vi "PositionReceiverAngleAttacker.vi"(6 "AnguloGol":dbl, 8 "error in (no error)":errorcluster, 9 "atacando contra":bool, 10 "Game":refnum<class "Game.lvclass">, 11 "PositionToReceivePassSkill in":refnum<class "PositionToReceivePassSkill.lvclass">) -> (0 "error out":errorcluster, 1 "AttackerPositive?":bool, 2 "theta final":dbl, 3 "PositionToReceivePassSkill out":refnum<class "PositionToReceivePassSkill.lvclass">, 4 "YdoAttacker 2":dbl, 5 "XdoAttacker 2":dbl)   [LabVIEW 2018, in "PositionToReceivePassSkill.lvclass"]
uses:
  PositionToReceivePassSkill.lvclass
  Game_class/Game.lvclass
  Game_class/Game.lvclass/Game.ctl
  Team_class/Team.lvclass/Team.ctl
  Robot_class/roles.ctl
  Robot_class/Robot.lvclass/Robot.ctl
  Object_class/Object.lvclass/Object.ctl
  Robot_class/Read role.vi
  Object_class/Read x.vi
  Object_class/Read y.vi
  Robot_class/Read id.vi
  Game_class/Read OffensiveTeam.vi
  Game_class/Read EnemyRef.vi
  Game_class/Read FieldRef.vi
  Team_class/Read RobotRef.vi
  Enemy_class/Enemy.lvclass
  Ally_class/Ally.lvclass
  Robot_class/Robot.lvclass
  Field_class/Field.lvclass
panel:
  in  "valor de theta 3":dbl
  in  "tamanho do intervalo 3":dbl
  in  "inicio do intervalo 3":dbl
  in  "fim do intervalo 3":dbl
  in  "Contador 4":dbl
  in  "Array 3":dbl[](array[numeric])=[0.0, 0.0, 0.0, 0.0, 0.0, 0.0]
  in  "valor de theta 2":dbl
  in  "tamanho do intervalo 2":dbl
  in  "inicio do intervalo 2":dbl
  in  "fim do intervalo 2":dbl
  in  "Contador 3":dbl
  in  "Array 2":dbl[](array[numeric])=[0.0, 0.0, 0.0, 0.0, 0.0, 0.0]
  in  "XdoAttacker":dbl
  in  "YdoAttacker":dbl
  in  "RobôsParaAnalisar":dbl[][](array[numeric])=[[99999.0, 99999.0], [99999.0, 99999.0], [99999.0, 99999.0], [99999.0, 99999.0], [99999.0, 99999.0], [99999.0, 99999.0], [99999.0, 99999.0]]
  in  "Contador":dbl
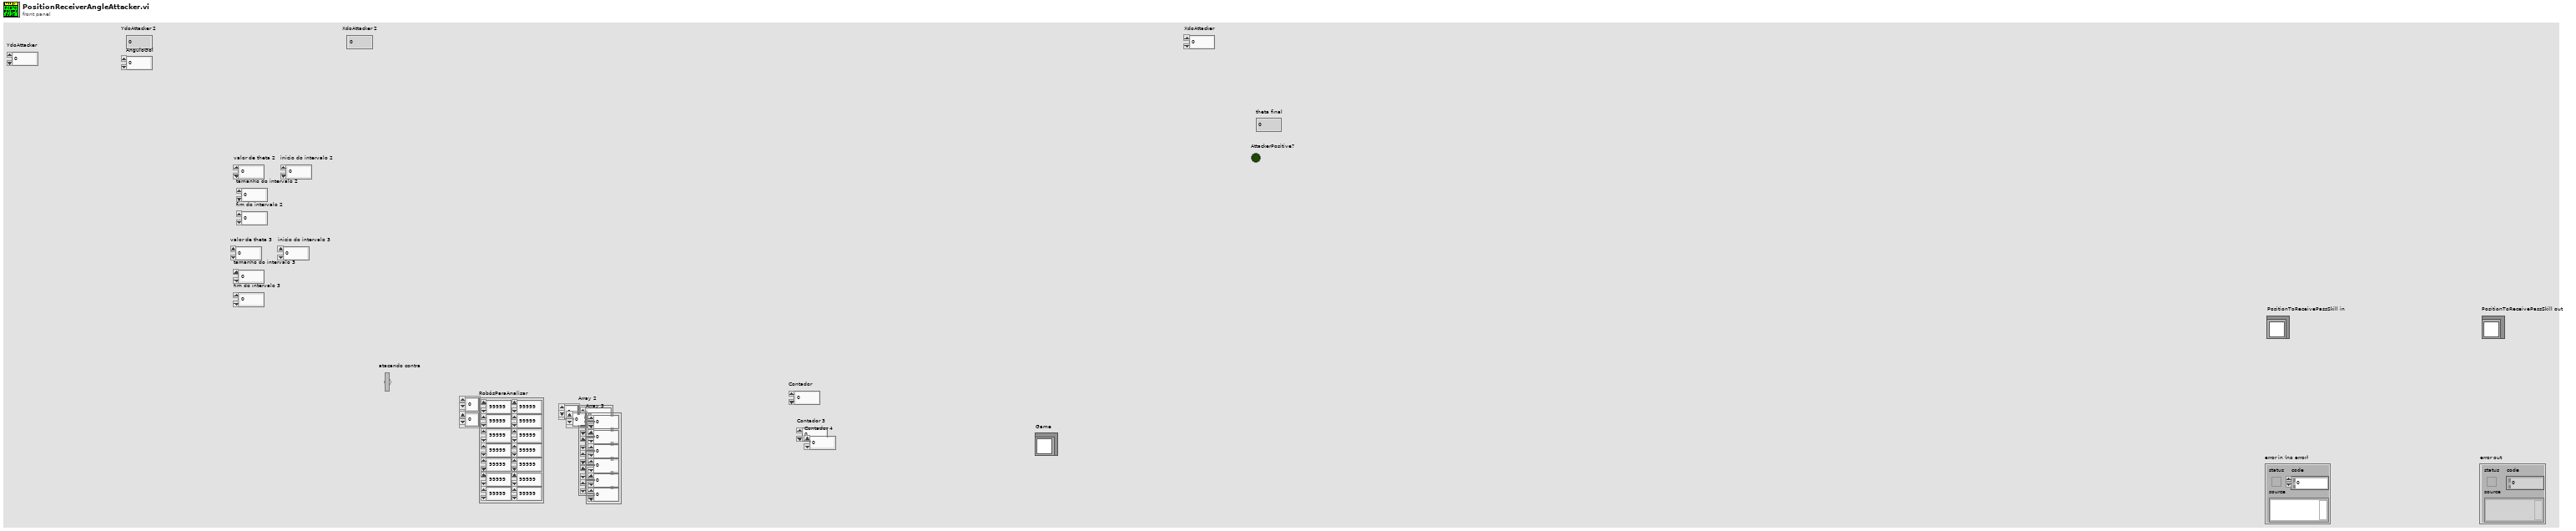
[diagram p1: front panel]
types:
  T1 = typedef "roles.ctl" = enum16{"PenaltyDefense", "PreparePassReceiver", "PassObserver", "Timeout", "Goto", "ZigZag", "None", "BallOutOfField", "DefenderArea", "Duelist", "AttackerStop", "FollowAttacker", "KeeperRole", "KickPenalty", "AttackerAimGoal", "AttackerBlock", "Marker", "Halt", "Shoot", "PassKicker", "PassReceiver", "TestRole", "PenaltyAttacker"}
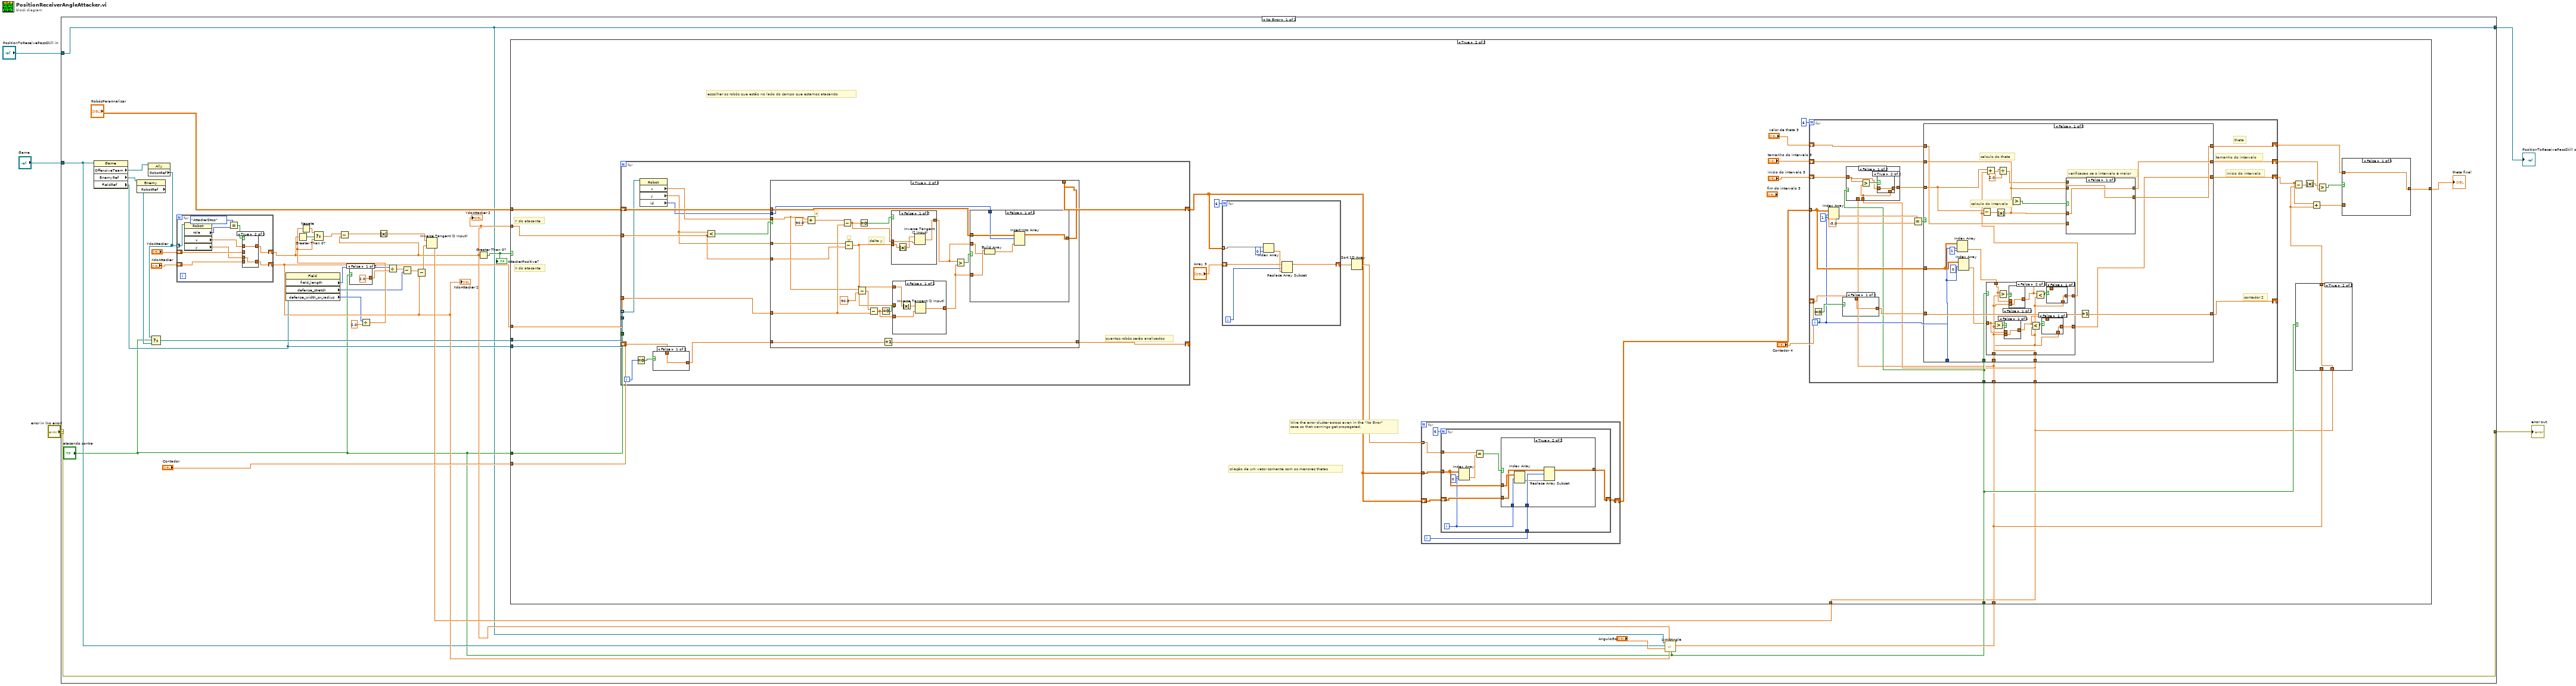
[diagram p0: block diagram]
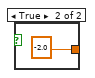
[diagram p2: hidden frame]
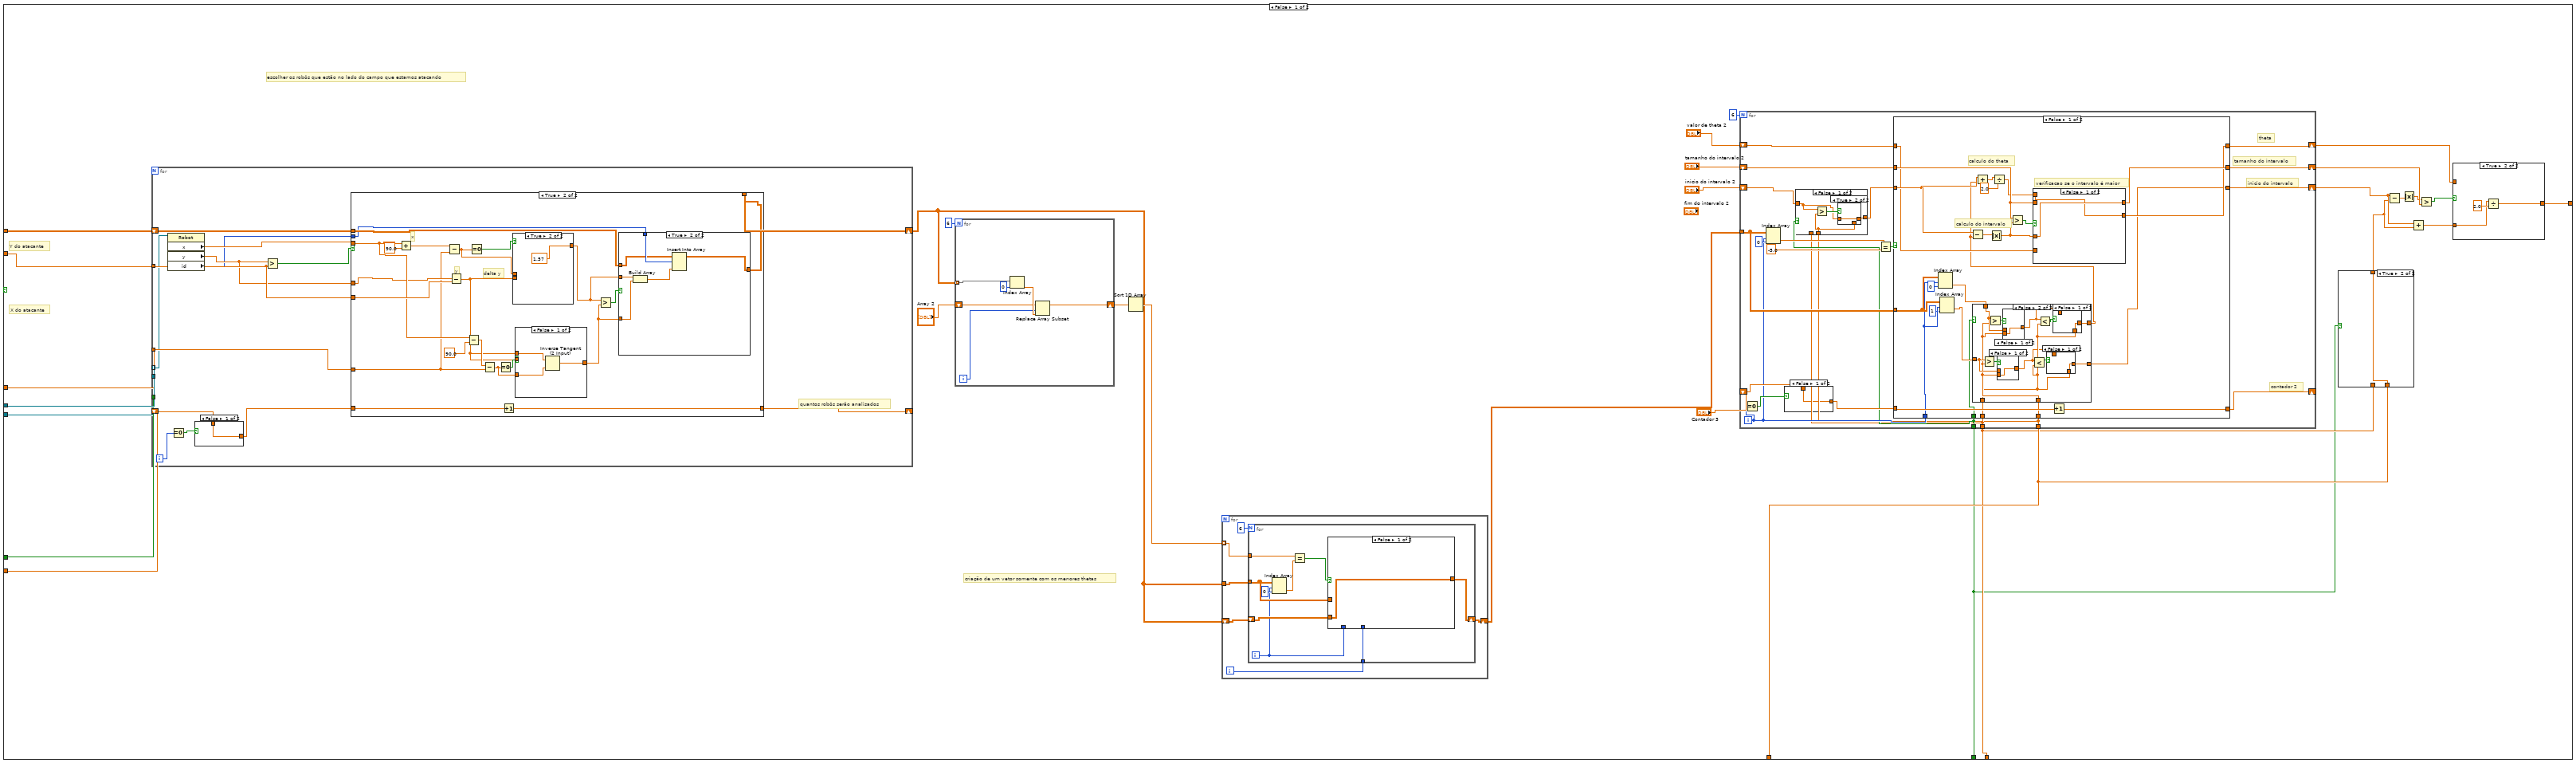
[diagram p3: hidden frame]
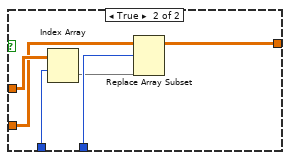
[diagram p6: hidden frame]
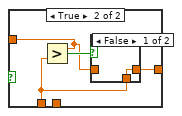
[diagram p8: hidden frame]
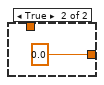
[diagram p10: hidden frame]
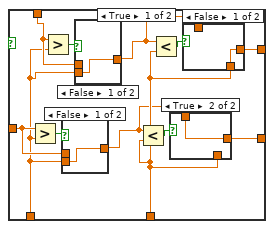
[diagram p11: hidden frame]
diagram:
  n1 = case shown="No Error" "error in (no error)" {
    selector: "error in (no error)" -> [w40 w525]
    tunnel: [w40 w525] -> w4
    tunnel: [w6 w524] -> w2
    tunnel: "PositionToReceivePassSkill in" -> [w6 w524]
    tunnel: "Game" -> [w8 _]
    frame No Error {
      # "Wire the error cluster across even in the \"No Error\"\ncase so that warnings get propagated."
      n2 = property class="Game"(reference=w8) -> ("OffensiveTeam"=w16:refnum<class "Ally.lvclass">, "EnemyRef"=w14:refnum<class "Enemy.lvclass">, "FieldRef"=w12:refnum<class "Field.lvclass">)  [unwired: 1 in, 2 out]
      n3 = property class="Enemy"(reference=w14) -> ("RobotRef"=w13:refnum<class "Robot.lvclass">[])  [unwired: 1 in, 2 out]
      n4 = property class="Ally"(reference=w16) -> ("RobotRef"=w15:refnum<class "Robot.lvclass">[])  [unwired: 1 in, 2 out]
      n5 = Select(t=w15, s="atacando contra", f=w13) -> (s? t:f=w39:refnum<class "Robot.lvclass">[])
      n6 = for {
        tunnel: w15 -> [w514] mode=indexing
        shift-right: [w518] -> w24
        shift-left: "YdoAttacker" -> [w517]
        shift-right: [w515] -> w21
        shift-left: "XdoAttacker" -> [w516]
        n7 = property class="Robot"(reference=w514) -> ("role"=w511:T1, "x"=w512:dbl, "y"=w513:dbl)  [unwired: 1 in, 2 out]
        n8 = Equal?(x=roles."AttackerStop", y=w511) -> (x = y?=w519:bool)
        n9 = case shown="True" w519 {
          tunnel: w512 -> [_ w523]
          tunnel: [w521 w523] -> w518
          tunnel: w517 -> [w521 _]
          tunnel: w513 -> [_ w522]
          tunnel: w516 -> [w520 _]
          tunnel: [w520 w522] -> w515
          frame False {
          }
          frame True {
          }
        }
      }
      "YdoAttacker 2" <- w24
      "XdoAttacker 2" <- w21
      n10 = property class="Field"(reference=w12) -> ("field_length"=w11:i32, "defense_stretch"=w10:i32, "defense_width_or_radius"=w9:i32)  [unwired: 1 in, 2 out]
      n11 = Greater Than 0?(x=w24) -> (x > 0?=w32:bool)
      n12 = case shown="False" "atacando contra" {
        tunnel: [2.0 ("y") -2.0 ("y")] -> w30
        frame False {
        }
        frame True {
        }
      }
      n13 = Divide(x=w9, y=2.0) -> (x/y=w28:dbl)
      n14 = Negate(x=w28) -> (-x=w31:dbl)
      n15 = Select(t=w31, s=w32, f=w28) -> (s? t:f=w23:dbl)
      n16 = Subtract(x=w23, y=w24) -> (x-y=w20:dbl)
      n17 = Absolute Value(x=w20) -> (abs(x)=w19:dbl)
      n18 = Divide(x=w11, y=w30) -> (x/y=w18:dbl)
      n19 = Subtract(x=w18, y=w10) -> (x-y=w17:dbl)
      n20 = Subtract(x=w17, y=w21) -> (x-y=w22:dbl)
      n21 = Inverse Tangent (2 Input)(1:w22, 2:w19) -> (0:w27:dbl)
      n22 = Greater Than 0?(x=w24) -> (x > 0?=w33:bool)
      "AttackerPositive?" <- w33
      n23 = call-dynamic "LimitAngle.vi"("atacando contra"="atacando contra", "XdoAttacker"=w21, "YdoAttacker"=w24, "AnguloGol"="AnguloGol", "Game"=w8, "PositionToReceivePassSkill in"=w6) -> ("Angulo Limite"=w25:dbl)  [unwired: 3 in, 2 out]
      n24 = case shown="True" w33 {
        tunnel: w39 -> [w72 w305]
        tunnel: "atacando contra" -> [w71 w304]
        tunnel: "Contador" -> [w70 w303]
        tunnel: "RobôsParaAnalisar" -> [w69 w302]
        tunnel: w12 -> [w68 w301]
        tunnel: [w54 w287] -> w36
        tunnel: w24 -> [w48 w281]
        tunnel: w21 -> [w47 w280]
        tunnel: w27 -> [w45 w276]
        tunnel: "atacando contra" -> [w43 w279]
        tunnel: w25 -> [w44 w278]
        frame False {
          # "X do atacante"
          # "Y do atacante"
          # "criação de um vetor somente com os menores thetas"
          # "escolher os robôs que estão no lado do campo que estamos atacando"
          n25 = for {
            tunnel: w72 -> [w216] mode=indexing
            tunnel: w71 -> [_]
            shift-right: [w220] -> w58
            shift-left: w69 -> [w226]
            shift-right: [w221] -> _
            shift-left: w70 -> [w223]
            tunnel: w68 -> [_]
            tunnel: w48 -> [w218]
            tunnel: w47 -> [w217]
            i -> [w224]
            # "quantos robôs serão analisados"
            n26 = property class="Robot"(reference=w216) -> ("x"=w215:dbl, "y"=w214:dbl, "id"=w213:i32)  [unwired: 1 in, 2 out]
            n27 = Equal To 0?(x=w224) -> (x = 0?=w225:bool)
            n28 = case shown="False" w225 {
              tunnel: w223 -> [w227 _]
              tunnel: [w227 0.0] -> w222
              frame False {
              }
              frame True {
              }
            }
            n29 = Greater?(x=w214, y=w218) -> (0:w219:bool)
            n30 = case shown="True" w219 {
              tunnel: w226 -> [w233 w253]
              tunnel: w213 -> [w232 w252]
              tunnel: w215 -> [_ w243]
              tunnel: w214 -> [_ w242]
              tunnel: w222 -> [w234 w254]
              tunnel: [w234 w255] -> w221
              tunnel: [w229 w251] -> w220
              tunnel: w218 -> [_ w244]
              tunnel: w217 -> [_ w240]
              frame False {
                w231 = -5.0 ("element")
                n31 = Build Array(w231, w231) -> (w230:dbl[])
                n32 = Insert Into Array(array=w233, index (row)=w232, new element=w230) -> (w229:dbl[][])  [unwired: 1 in]
              }
              frame True {
                # "delta y"
                # "y"
                # "x"
                n33 = Add(x=w243, y=90.0) -> (x+y=w241:dbl)
                n34 = Subtract(x=w241, y=w240) -> (x-y=w238:dbl)
                n35 = Subtract(x=w242, y=w244) -> (x-y=w235:dbl)
                n36 = Subtract(x=w243, y=90.0) -> (x-y=w248:dbl)
                n37 = Equal To 0?(x=w238) -> (x = 0?=w239:bool)
                n38 = Subtract(x=w248, y=w240) -> (x-y=w236:dbl)
                n39 = Equal To 0?(x=w236) -> (x = 0?=w237:bool)
                n40 = Increment(x=w254) -> (x+1=w255:dbl)
                n41 = case shown="True" w239 {
                  tunnel: [w273 1.57] -> w246
                  tunnel: w235 -> [w274 _]
                  tunnel: w238 -> [w272 _]
                  frame False {
                    n42 = Inverse Tangent (2 Input)(1:w272, 2:w274) -> (0:w273:dbl)
                  }
                  frame True {
                  }
                }
                n43 = case shown="False" w237 {
                  tunnel: [w258 1.57] -> w245
                  tunnel: w235 -> [_ _]
                  tunnel: w236 -> [w257 _]
                  tunnel: w235 -> [w256 _]
                  frame False {
                    n44 = Inverse Tangent (2 Input)(1:w257, 2:w256) -> (0:w258:dbl)
                  }
                  frame True {
                  }
                }
                n45 = Greater?(x=w246, y=w245) -> (0:w247:bool)
                n46 = case shown="True" w247 {
                  tunnel: w253 -> [w262 w268]
                  tunnel: w252 -> [w264 w271]
                  tunnel: w246 -> [w261 w269]
                  tunnel: w245 -> [w263 w267]
                  tunnel: [w260 w266] -> w251
                  frame False {
                    n47 = Build Array(w263, w261) -> (w265:dbl[])
                    n48 = Insert Into Array(array=w262, index (row)=w264, new element=w265) -> (w260:dbl[][])  [unwired: 1 in]
                  }
                  frame True {
                    n49 = Build Array(w269, w267) -> (w270:dbl[])
                    n50 = Insert Into Array(array=w268, index (row)=w271, new element=w270) -> (w266:dbl[][])  [unwired: 1 in]
                  }
                }
              }
            }
          }
          n51 = for {
            N: 6 -> [_]
            tunnel: w58 -> [w106] mode=indexing
            shift-right: [w101] -> w60
            shift-left: "Array 2" -> [w102]
            i -> [w103]
            n52 = Index Array(array=w106, index=0) -> (element=w104:dbl)
            n53 = Replace Array Subset(array=w102, new element=w104, index=w103) -> (w101:dbl[])
          }
          n54 = Sort 1D Array(array=w60) -> (sorted array=w59:dbl[])
          n55 = for {
            tunnel: w59 -> [w81] mode=indexing
            tunnel: w58 -> [w83]
            shift-right: [w79] -> w57
            shift-left: w58 -> [w82]
            i -> [w80]
            n56 = for {
              N: 6 -> [_]
              tunnel: w83 -> [w89]
              shift-right: [w85] -> w79
              shift-left: w82 -> [w88]
              tunnel: w81 -> [w91]
              tunnel: w80 -> [w86]
              i -> [w87]
              n57 = Index Array(array=w89, index (row)=w87, index (col)=0 ("disabled index (col)")) -> (element=w92:dbl)
              n58 = Equal?(x=w91, y=w92) -> (x = y?=w90:bool)
              n59 = case shown="False" w90 {
                tunnel: w89 -> [_ w100]
                tunnel: w88 -> [w94 w96]
                tunnel: w87 -> [_ w99]
                tunnel: w86 -> [_ w98]
                tunnel: [w94 w95] -> w85
                frame False {
                }
                frame True {
                  n60 = Index Array(array=w100, index (row)=w99) -> (element=w97:dbl[])  [unwired: 1 in]
                  n61 = Replace Array Subset(array=w96, new element=w97, index (row)=w98) -> (w95:dbl[][])  [unwired: 1 in]
                }
              }
            }
          }
          n62 = for {
            N: 6 -> [_]
            tunnel: w57 -> [w113]
            shift-right: [w121] -> w53
            shift-left: "valor de theta 2" -> [w122]
            shift-right: [w119] -> w56
            shift-left: "tamanho do intervalo 2" -> [w120]
            shift-right: [w118] -> w50
            shift-left: "inicio do intervalo 2" -> [w110]
            shift-right: [w114] -> _
            shift-left: "Contador 3" -> [w116]
            tunnel: w44 -> [w108]
            tunnel: w45 -> [w107]
            tunnel: w43 -> [w111]
            i -> [w112]
            # "contador 2"
            # "inicio do intervalo"
            # "tamanho do intervalo"
            # "theta"
            n63 = Equal To 0?(x=w112) -> (x = 0?=w117:bool)
            n64 = Index Array(array=w113, index (row)=w112, index (col)=0 ("disabled index (col)")) -> (element=w124:dbl)
            n65 = case shown="False" w117 {
              tunnel: w116 -> [w139 _]
              tunnel: [w139 0.0] -> w115
              frame False {
              }
              frame True {
              }
            }
            n66 = case shown="False" w111 {
              tunnel: w108 -> [_ w133]
              tunnel: w110 -> [w129 w134]
              tunnel: [w127 w135] -> w109
              tunnel: w107 -> [w128 _]
              frame False {
                n67 = Greater?(x=w129, y=w128) -> (0:w130:bool)
                n68 = case shown="True" w130 {
                  tunnel: [w131 w132] -> w127
                  tunnel: w129 -> [_ w132]
                  tunnel: w128 -> [w131 _]
                  frame False {
                  }
                  frame True {
                  }
                }
              }
              frame True {
                n69 = Greater?(x=w134, y=w133) -> (0:w136:bool)
                n70 = case shown="False" w136 {
                  tunnel: [w137 w138] -> w135
                  tunnel: w134 -> [_ w138]
                  tunnel: w133 -> [w137 _]
                  frame False {
                  }
                  frame True {
                  }
                }
              }
            }
            n71 = Equal?(x=w124, y=-5.0) -> (x = y?=w125:bool)
            n72 = case shown="False" w125 {
              tunnel: w122 -> [w148 w212]
              tunnel: [w149 w212] -> w121
              tunnel: w120 -> [w153 w211]
              tunnel: [w152 w211] -> w119
              tunnel: w109 -> [w164 w210]
              tunnel: [w146 w210] -> w118
              tunnel: w115 -> [w162 w209]
              tunnel: [w163 w209] -> w114
              tunnel: w113 -> [w161 _]
              tunnel: w112 -> [w160 _]
              tunnel: w108 -> [w143 _]
              tunnel: w107 -> [w142 _]
              tunnel: w111 -> [w141 _]
              frame False {
                # "calculo do theta"
                # "calculo do intervalo"
                # "verificacao se o intervalo é maior"
                n73 = Index Array(array=w161, index (row)=w160, index (col)=0 ("disabled index (col)")) -> (element=w145:dbl)
                n74 = Index Array(array=w161, index (row)=w160, index (col)=1 ("disabled index (col)")) -> (element=w147:dbl)
                n75 = case shown="False" w141 {
                  tunnel: w143 -> [w168 w186]
                  tunnel: w145 -> [w175 w195]
                  tunnel: w142 -> [w167 w187]
                  tunnel: [w173 w193] -> w144
                  tunnel: w147 -> [w169 w189]
                  tunnel: [w166 w188] -> w146
                  frame True {
                    n76 = Greater?(x=w169, y=w168) -> (0:w171:bool)
                    n77 = Greater?(x=w175, y=w168) -> (0:w176:bool)
                    n78 = case shown="False" w171 {
                      tunnel: [w179 w180] -> w165
                      tunnel: w169 -> [_ w180]
                      tunnel: w168 -> [w179 _]
                      frame False {
                      }
                      frame True {
                      }
                    }
                    n79 = case shown="False" w176 {
                      tunnel: [w183 w184] -> w172
                      tunnel: w175 -> [_ w184]
                      tunnel: w168 -> [w183 _]
                      frame False {
                      }
                      frame True {
                      }
                    }
                    n80 = Less?(x=w165, y=w167) -> (x < y?=w170:bool)
                    n81 = Less?(x=w172, y=w167) -> (x < y?=w174:bool)
                    n82 = case shown="True" w170 {
                      tunnel: [w177 w178] -> w166
                      tunnel: w165 -> [_ w178]
                      tunnel: w167 -> [w177 _]
                      frame False {
                      }
                      frame True {
                      }
                    }
                    n83 = case shown="False" w174 {
                      tunnel: [w181 w182] -> w173
                      tunnel: w172 -> [_ w182]
                      tunnel: w167 -> [w181 _]
                      frame False {
                      }
                      frame True {
                      }
                    }
                  }
                  frame False {
                    n84 = Greater?(x=w189, y=w187) -> (0:w191:bool)
                    n85 = Greater?(x=w195, y=w187) -> (0:w196:bool)
                    n86 = case shown="False" w191 {
                      tunnel: [w199 w200] -> w185
                      tunnel: w189 -> [_ w200]
                      tunnel: w187 -> [w199 _]
                      frame False {
                      }
                      frame True {
                      }
                    }
                    n87 = case shown="False" w196 {
                      tunnel: [w203 w204] -> w192
                      tunnel: w195 -> [_ w204]
                      tunnel: w187 -> [w203 _]
                      frame False {
                      }
                      frame True {
                      }
                    }
                    n88 = Less?(x=w185, y=w186) -> (x < y?=w190:bool)
                    n89 = Less?(x=w192, y=w186) -> (x < y?=w194:bool)
                    n90 = case shown="False" w190 {
                      tunnel: [w197 w198] -> w188
                      tunnel: w185 -> [_ w198]
                      tunnel: w186 -> [w197 _]
                      frame False {
                      }
                      frame True {
                      }
                    }
                    n91 = case shown="False" w194 {
                      tunnel: [w201 w202] -> w193
                      tunnel: w192 -> [_ w202]
                      tunnel: w186 -> [w201 _]
                      frame False {
                      }
                      frame True {
                      }
                    }
                  }
                }
                n92 = Subtract(x=w164, y=w144) -> (x-y=w157:dbl)
                n93 = Add(x=w164, y=w144) -> (x+y=w156:dbl)
                n94 = Absolute Value(x=w157) -> (abs(x)=w151:dbl)
                n95 = Divide(x=w156, y=2.0) -> (x/y=w150:dbl)
                n96 = Greater?(x=w153, y=w151) -> (0:w154:bool)
                n97 = case shown="False" w154 {
                  tunnel: w153 -> [_ w208]
                  tunnel: [w206 w208] -> w152
                  tunnel: w151 -> [w206 _]
                  tunnel: w148 -> [_ w207]
                  tunnel: w150 -> [w205 _]
                  tunnel: [w205 w207] -> w149
                  frame False {
                  }
                  frame True {
                  }
                }
                n98 = Increment(x=w162) -> (x+1=w163:dbl)
              }
              frame True {
              }
            }
          }
          n99 = case shown="True" w43 {
            tunnel: w44 -> [w73 _]
            tunnel: [w73 w74] -> w46
            tunnel: w45 -> [_ w74]
            frame False {
            }
            frame True {
            }
          }
          n100 = Subtract(x=w50, y=w46) -> (x-y=w52:dbl)
          n101 = Absolute Value(x=w52) -> (abs(x)=w51:dbl)
          n102 = Add(x=w50, y=w46) -> (x+y=w49:dbl)
          n103 = Greater?(x=w51, y=w56) -> (0:w55:bool)
          n104 = case shown="True" w55 {
            tunnel: [w75 w77] -> w54
            tunnel: w53 -> [w75 _]
            tunnel: w49 -> [_ w76]
            frame False {
            }
            frame True {
              n105 = Divide(x=w76, y=2.0) -> (x/y=w77:dbl)
            }
          }
        }
        frame True {
          # "X do atacante"
          # "Y do atacante"
          # "criação de um vetor somente com os menores thetas"
          # "escolher os robôs que estão no lado do campo que estamos atacando"
          n106 = for {
            tunnel: w305 -> [w449] mode=indexing
            tunnel: w304 -> [_]
            shift-right: [w453] -> w291
            shift-left: w302 -> [w459]
            shift-right: [w454] -> _
            shift-left: w303 -> [w456]
            tunnel: w301 -> [_]
            tunnel: w281 -> [w451]
            tunnel: w280 -> [w450]
            i -> [w457]
            # "quantos robôs serão analisados"
            n107 = Equal To 0?(x=w457) -> (x = 0?=w458:bool)
            n108 = property class="Robot"(reference=w449) -> ("x"=w448:dbl, "y"=w446:dbl, "id"=w447:i32)  [unwired: 1 in, 2 out]
            n109 = case shown="False" w458 {
              tunnel: w456 -> [w460 _]
              tunnel: [w460 0.0] -> w455
              frame False {
              }
              frame True {
              }
            }
            n110 = Less?(x=w446, y=w451) -> (x < y?=w452:bool)
            n111 = case shown="True" w452 {
              tunnel: w459 -> [w465 w485]
              tunnel: w447 -> [_ w484]
              tunnel: w448 -> [_ w467]
              tunnel: w455 -> [w466 w486]
              tunnel: [w466 w487] -> w454
              tunnel: [w462 w483] -> w453
              tunnel: w451 -> [_ w476]
              tunnel: w450 -> [_ w474]
              tunnel: w446 -> [_ w468]
              frame False {
                w464 = -5.0 ("element")
                n112 = Build Array(w464, w464) -> (w463:dbl[])
                n113 = Insert Into Array(array=w465, new element=w463) -> (w462:dbl[][])  [unwired: 2 in]
              }
              frame True {
                # "delta y"
                # "y"
                # "x"
                n114 = Add(x=w467, y=90.0) -> (x+y=w475:dbl)
                n115 = Subtract(x=w475, y=w474) -> (x-y=w472:dbl)
                n116 = Subtract(x=w468, y=w476) -> (x-y=w469:dbl)
                n117 = Subtract(x=w467, y=90.0) -> (x-y=w480:dbl)
                n118 = Equal To 0?(x=w472) -> (x = 0?=w473:bool)
                n119 = Subtract(x=w480, y=w474) -> (x-y=w470:dbl)
                n120 = Equal To 0?(x=w470) -> (x = 0?=w471:bool)
                n121 = Increment(x=w486) -> (x+1=w487:dbl)
                n122 = case shown="False" w473 {
                  tunnel: [w508 1.57] -> w478
                  tunnel: w469 -> [w506 _]
                  tunnel: w472 -> [w507 _]
                  frame False {
                    n123 = Absolute Value(x=w506) -> (abs(x)=w505:dbl)
                    n124 = Inverse Tangent (2 Input)(1:w507, 2:w505) -> (0:w508:dbl)
                  }
                  frame True {
                  }
                }
                n125 = case shown="False" w471 {
                  tunnel: [w491 1.57] -> w477
                  tunnel: w469 -> [_ _]
                  tunnel: w470 -> [w490 _]
                  tunnel: w469 -> [w488 _]
                  frame False {
                    n126 = Absolute Value(x=w488) -> (abs(x)=w489:dbl)
                    n127 = Inverse Tangent (2 Input)(1:w490, 2:w489) -> (0:w491:dbl)
                  }
                  frame True {
                  }
                }
                n128 = Greater?(x=w478, y=w477) -> (0:w479:bool)
                n129 = case shown="False" w479 {
                  tunnel: w485 -> [w496 w502]
                  tunnel: w484 -> [w493 w499]
                  tunnel: w478 -> [w495 w503]
                  tunnel: w477 -> [w497 w501]
                  tunnel: [w494 w500] -> w483
                  frame False {
                    n130 = Build Array(w497, w495) -> (w498:dbl[])
                    n131 = Insert Into Array(array=w496, index (row)=w493, new element=w498) -> (w494:dbl[][])  [unwired: 1 in]
                  }
                  frame True {
                    n132 = Build Array(w503, w501) -> (w504:dbl[])
                    n133 = Insert Into Array(array=w502, index (row)=w499, new element=w504) -> (w500:dbl[][])  [unwired: 1 in]
                  }
                }
              }
            }
          }
          n134 = for {
            N: 6 -> [_]
            tunnel: w291 -> [w339] mode=indexing
            shift-right: [w334] -> w293
            shift-left: "Array 3" -> [w335]
            i -> [w336]
            n135 = Index Array(array=w339, index=0) -> (element=w337:dbl)
            n136 = Replace Array Subset(array=w335, new element=w337, index=w336) -> (w334:dbl[])
          }
          n137 = Sort 1D Array(array=w293) -> (sorted array=w292:dbl[])
          n138 = for {
            tunnel: w292 -> [w314] mode=indexing
            tunnel: w291 -> [w316]
            shift-right: [w312] -> w290
            shift-left: w291 -> [w315]
            i -> [w313]
            n139 = for {
              N: 6 -> [_]
              tunnel: w316 -> [w322]
              shift-right: [w318] -> w312
              shift-left: w315 -> [w321]
              tunnel: w314 -> [w324]
              tunnel: w313 -> [w319]
              i -> [w320]
              n140 = Index Array(array=w322, index (row)=w320, index (col)=0 ("disabled index (col)")) -> (element=w325:dbl)
              n141 = Equal?(x=w324, y=w325) -> (x = y?=w323:bool)
              n142 = case shown="True" w323 {
                tunnel: w322 -> [_ w333]
                tunnel: w321 -> [w327 w329]
                tunnel: w320 -> [_ w332]
                tunnel: w319 -> [_ w331]
                tunnel: [w327 w328] -> w318
                frame False {
                }
                frame True {
                  n143 = Index Array(array=w333, index (row)=w332) -> (element=w330:dbl[])  [unwired: 1 in]
                  n144 = Replace Array Subset(array=w329, new element=w330, index (row)=w331) -> (w328:dbl[][])  [unwired: 1 in]
                }
              }
            }
          }
          n145 = for {
            N: 6 -> [_]
            tunnel: w290 -> [w346]
            shift-right: [w354] -> w286
            shift-left: "valor de theta 3" -> [w355]
            shift-right: [w352] -> w289
            shift-left: "tamanho do intervalo 3" -> [w353]
            shift-right: [w351] -> w283
            shift-left: "inicio do intervalo 3" -> [w342]
            shift-right: [w347] -> _
            shift-left: "Contador 4" -> [w349]
            tunnel: w279 -> [w344]
            tunnel: w278 -> [w343]
            tunnel: w276 -> [w340]
            i -> [w345]
            # "contador 2"
            # "inicio do intervalo"
            # "tamanho do intervalo"
            # "theta"
            n146 = Equal To 0?(x=w345) -> (x = 0?=w350:bool)
            n147 = Index Array(array=w346, index (row)=w345, index (col)=1 ("disabled index (col)")) -> (element=w357:dbl)
            n148 = case shown="False" w350 {
              tunnel: w349 -> [w372 _]
              tunnel: [w372 0.0] -> w348
              frame False {
              }
              frame True {
              }
            }
            n149 = case shown="False" w344 {
              tunnel: w343 -> [_ w366]
              tunnel: w342 -> [w362 w367]
              tunnel: [w360 w368] -> w341
              tunnel: w340 -> [w361 _]
              frame False {
                n150 = Greater?(x=w362, y=w361) -> (0:w363:bool)
                n151 = case shown="True" w363 {
                  tunnel: [w364 w365] -> w360
                  tunnel: w362 -> [_ w365]
                  tunnel: w361 -> [w364 _]
                  frame False {
                  }
                  frame True {
                  }
                }
              }
              frame True {
                n152 = Greater?(x=w367, y=w366) -> (0:w369:bool)
                n153 = case shown="False" w369 {
                  tunnel: [w370 w371] -> w368
                  tunnel: w367 -> [_ w371]
                  tunnel: w366 -> [w370 _]
                  frame False {
                  }
                  frame True {
                  }
                }
              }
            }
            n154 = Equal?(x=w357, y=-5.0) -> (x = y?=w358:bool)
            n155 = case shown="False" w358 {
              tunnel: w355 -> [w382 w445]
              tunnel: [w383 w445] -> w354
              tunnel: w353 -> [w387 w444]
              tunnel: [w386 w444] -> w352
              tunnel: [w376 w442] -> w351
              tunnel: w348 -> [w396 w443]
              tunnel: [w397 w443] -> w347
              tunnel: w346 -> [w395 _]
              tunnel: w345 -> [w394 _]
              tunnel: w344 -> [w381 _]
              tunnel: w343 -> [w380 _]
              tunnel: w340 -> [w379 _]
              tunnel: w341 -> [w375 w442]
              frame False {
                # "calculo do theta"
                # "calculo do intervalo"
                # "verificacao se o intervalo é maior"
                n156 = Index Array(array=w395, index (row)=w394, index (col)=1 ("disabled index (col)")) -> (element=w374:dbl)
                n157 = Index Array(array=w395, index (row)=w394, index (col)=0 ("disabled index (col)")) -> (element=w377:dbl)
                n158 = case shown="False" w381 {
                  tunnel: w380 -> [w401 w419]
                  tunnel: w374 -> [w408 w428]
                  tunnel: w379 -> [w400 w420]
                  tunnel: [w406 w426] -> w378
                  tunnel: w377 -> [w402 w422]
                  tunnel: [w399 w421] -> w376
                  frame True {
                    n159 = Greater?(x=w402, y=w401) -> (0:w404:bool)
                    n160 = Greater?(x=w408, y=w401) -> (0:w409:bool)
                    n161 = case shown="False" w404 {
                      tunnel: [w412 w413] -> w398
                      tunnel: w402 -> [_ w413]
                      tunnel: w401 -> [w412 _]
                      frame False {
                      }
                      frame True {
                      }
                    }
                    n162 = case shown="False" w409 {
                      tunnel: [w416 w417] -> w405
                      tunnel: w408 -> [_ w417]
                      tunnel: w401 -> [w416 _]
                      frame False {
                      }
                      frame True {
                      }
                    }
                    n163 = Less?(x=w398, y=w400) -> (x < y?=w403:bool)
                    n164 = Less?(x=w405, y=w400) -> (x < y?=w407:bool)
                    n165 = case shown="True" w403 {
                      tunnel: [w410 w411] -> w399
                      tunnel: w398 -> [_ w411]
                      tunnel: w400 -> [w410 _]
                      frame False {
                      }
                      frame True {
                      }
                    }
                    n166 = case shown="False" w407 {
                      tunnel: [w414 w415] -> w406
                      tunnel: w405 -> [_ w415]
                      tunnel: w400 -> [w414 _]
                      frame False {
                      }
                      frame True {
                      }
                    }
                  }
                  frame False {
                    n167 = Greater?(x=w422, y=w420) -> (0:w424:bool)
                    n168 = Greater?(x=w428, y=w420) -> (0:w429:bool)
                    n169 = case shown="False" w424 {
                      tunnel: [w432 w433] -> w418
                      tunnel: w422 -> [_ w433]
                      tunnel: w420 -> [w432 _]
                      frame False {
                      }
                      frame True {
                      }
                    }
                    n170 = case shown="False" w429 {
                      tunnel: [w436 w437] -> w425
                      tunnel: w428 -> [_ w437]
                      tunnel: w420 -> [w436 _]
                      frame False {
                      }
                      frame True {
                      }
                    }
                    n171 = Less?(x=w418, y=w419) -> (x < y?=w423:bool)
                    n172 = Less?(x=w425, y=w419) -> (x < y?=w427:bool)
                    n173 = case shown="False" w423 {
                      tunnel: [w430 w431] -> w421
                      tunnel: w418 -> [_ w431]
                      tunnel: w419 -> [w430 _]
                      frame False {
                      }
                      frame True {
                      }
                    }
                    n174 = case shown="False" w427 {
                      tunnel: [w434 w435] -> w426
                      tunnel: w425 -> [_ w435]
                      tunnel: w419 -> [w434 _]
                      frame False {
                      }
                      frame True {
                      }
                    }
                  }
                }
                n175 = Subtract(x=w375, y=w378) -> (x-y=w391:dbl)
                n176 = Add(x=w375, y=w378) -> (x+y=w390:dbl)
                n177 = Absolute Value(x=w391) -> (abs(x)=w385:dbl)
                n178 = Divide(x=w390, y=2.0) -> (x/y=w384:dbl)
                n179 = Greater?(x=w387, y=w385) -> (0:w388:bool)
                n180 = case shown="False" w388 {
                  tunnel: w387 -> [_ w441]
                  tunnel: [w439 w441] -> w386
                  tunnel: w385 -> [w439 _]
                  tunnel: w382 -> [_ w440]
                  tunnel: w384 -> [w438 _]
                  tunnel: [w438 w440] -> w383
                  frame False {
                  }
                  frame True {
                  }
                }
                n181 = Increment(x=w396) -> (x+1=w397:dbl)
              }
              frame True {
              }
            }
          }
          n182 = case shown="True" w279 {
            tunnel: w278 -> [w306 _]
            tunnel: [w306 w307] -> w277
            tunnel: w276 -> [_ w307]
            frame False {
            }
            frame True {
            }
          }
          n183 = Subtract(x=w283, y=w277) -> (x-y=w285:dbl)
          n184 = Absolute Value(x=w285) -> (abs(x)=w284:dbl)
          n185 = Add(x=w283, y=w277) -> (x+y=w282:dbl)
          n186 = Greater?(x=w284, y=w289) -> (0:w288:bool)
          n187 = case shown="False" w288 {
            tunnel: [w308 w310] -> w287
            tunnel: w286 -> [w308 _]
            tunnel: w282 -> [_ w309]
            frame False {
            }
            frame True {
              n188 = Divide(x=w309, y=2.0) -> (x/y=w310:dbl)
            }
          }
        }
      }
      "theta final" <- w36
    }
    frame Error {
    }
  }
  "error out" <- w4
  "PositionToReceivePassSkill out" <- w2
